vi "Set All Minimum Log Level.vi"(8 "error in":errorcluster, 11 "log level":T1) -> (0 "error out":errorcluster)   [LabVIEW 2018, in "GLog.lvlib" / "Registry.lvlib"]
uses:
  Registry.lvlib
  api/Log Levels.ctl
  Registry Actions.ctl
  api/GLog.lvlib
panel:
  # "Connector Pane"
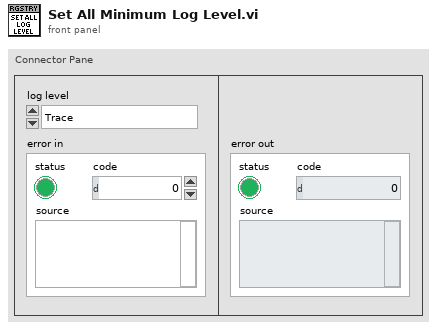
[diagram p1: front panel]
types:
  T1 = typedef "GLog.lvlib/Log Levels.ctl" = enum16{"Trace", "Debug", "Info", "Warning", "Error", "Critical"}
  T2 = typedef "GLog.lvlib/Registry.lvlib/Registry Actions.ctl" = enum16{"Register", "Log", "Enable", "Enable All", "Disable", "Disable All", "Get Enable State", "Get Minimum Log Level", "Set Minimum Log Level", "Set All Minimum Log Level", "Get Logger Info", "Get All Logger Info", "List", "Unregister", "Unregister All", "Shutdown"}
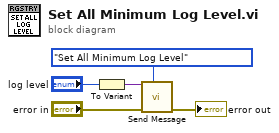
[diagram p0: block diagram]
diagram:
  n1 = To Variant(anything="log level") -> (Variant=w1:variant)
  n2 = call "Send Message.vi"("action"=Registry_Actions."Set All Minimum Log Level", "error in (no error)"="error in", "send data"=w1) -> ("error out"=→"error out":errorcluster)  [unwired: 7 in, 1 out]
